vi "Initialize Events.vi"(8 "error in":errorcluster) -> (0 "error out":errorcluster, 3 "Events":T1)   [LabVIEW 2019]
doc: "Initialize all user events.\n\n------------------\nJuan Navarro\nLab It Studio"
uses:
  Type Definitions/Events.ctl
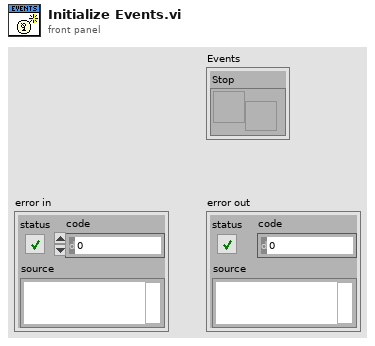
[diagram p1: front panel]
types:
  T1 = typedef "Events.ctl" = cluster{"Stop":refnum<user-event>}
  T2 = enum16{"Create Event", "Generate Event", "Destroy Event"}
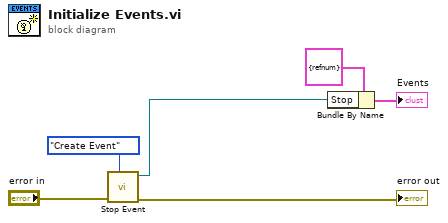
[diagram p0: block diagram]
diagram:
  n1 = call "Stop Event.vi"("Actions"=T2."Create Event", "error in"="error in") -> ("error out"=→"error out":errorcluster, "Stop"=w4:refnum<user-event>)  [unwired: 8 in]
  n2 = Bundle By Name(cluster=T1 {"Stop"=refnum} ("Events"), "Stop"=w4) -> (→"Events":T1)
